vi "ProjektKoncowy.vi"() -> ()   [LabVIEW 2022 SP3]
doc: "Use this template to build a standard state machine design pattern. Each state executes code and determines which state to transition to. Contrast this design pattern with the User Interface Event Handler pattern, in which code executes in response to user actions. Contrast this design pattern also with the Queued Message Handler pattern, in which each message handling code can queue zero or more new messages.\nNote: This template does not contain the most recent programming guidelines recommended by National Instruments. For a complete, project-based implementation of the Standard State Machine pattern, use the Create Project dialog box instead of this template."
uses:
  ProjektKoncowy.ctl
  <vilib>/numeric/Random Number (Range) DBL.vi
  <vilib>/Instr/_visa.llb/VISA Configure Serial Port (Instr).vi
panel:
  in  "Przeskok":dbl(slide)=2.9591836734693877 scale=0.0..10.0
  in  "Szerokosc sciezki":dbl(slide)=5.0 scale=0.0..10.0
  out "Wynik w Grze":dbl
  in  "Stop Button":bool
  out "Gra":waveform(dbl)[](graph)
  out "Dystans w cm":string
  # "Poziom Trudnosci"
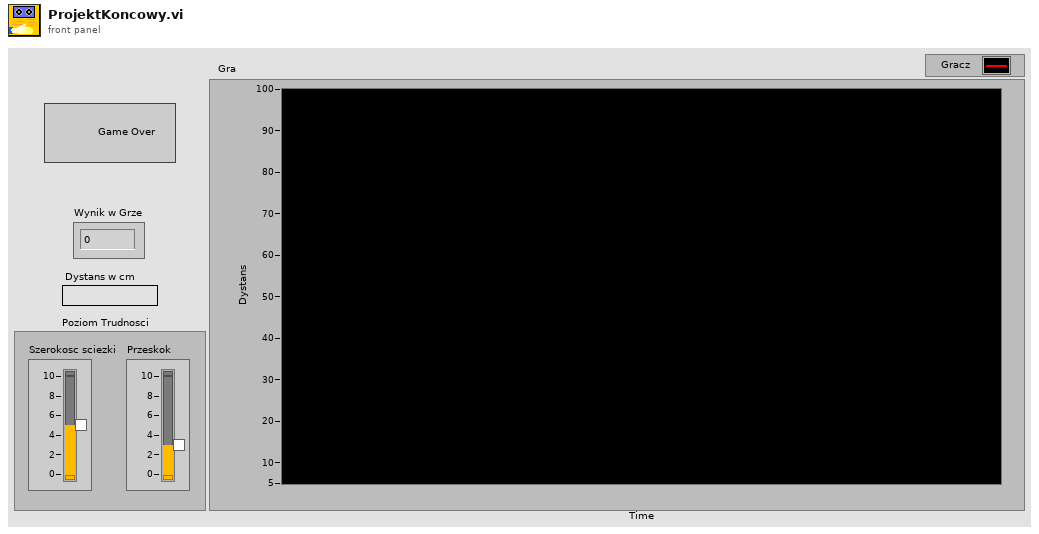
[diagram p1: front panel]
types:
  T1 = typedef "ProjektKoncowy.ctl" = enum16{"Rysuj", "Initialize", "Czytaj dystans", "Stop"}
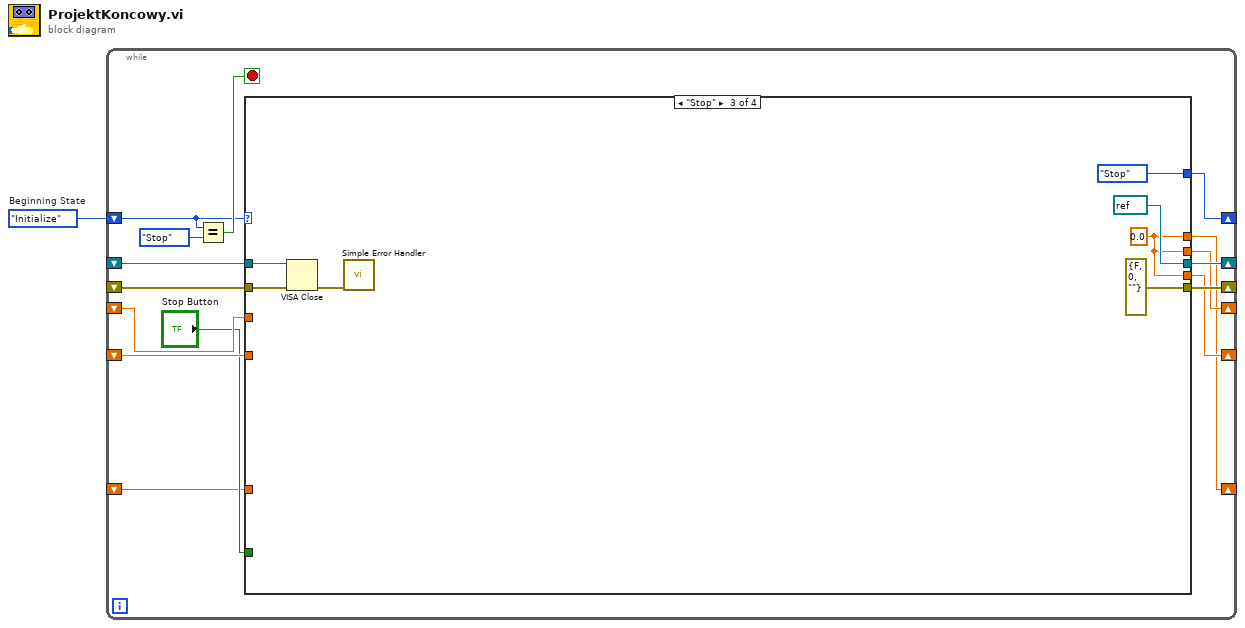
[diagram p0: block diagram]
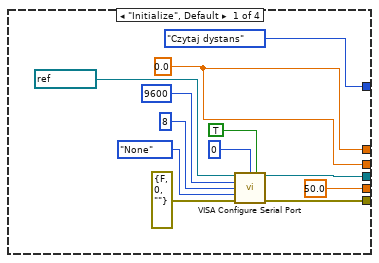
[diagram p2: hidden frame]
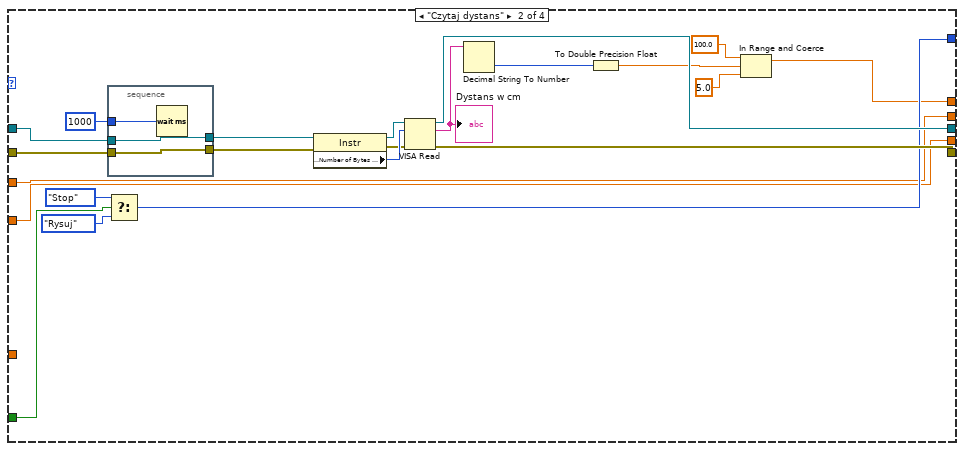
[diagram p3: hidden frame]
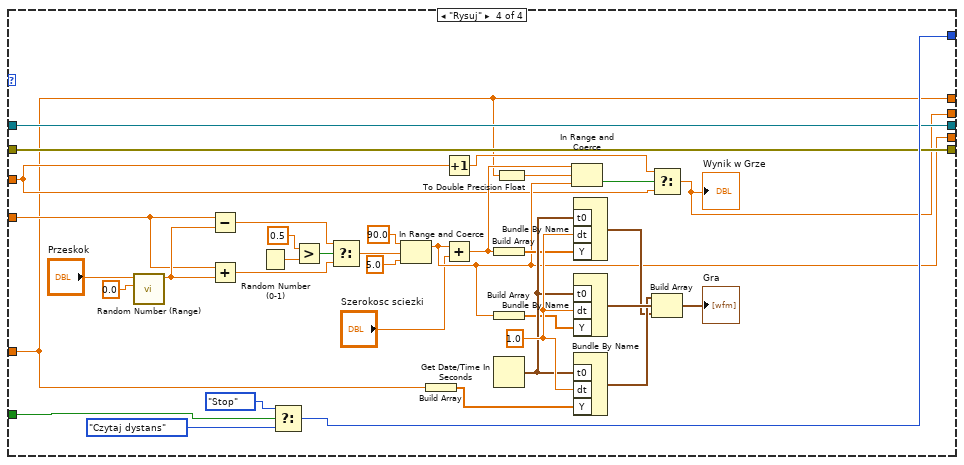
[diagram p4: hidden frame]
diagram:
  w1 = ProjektKoncowy."Initialize"  # Beginning State
  n1 = while {
    shift-right: [w13] -> _
    shift-left: w1 -> [w14]
    shift-right: [w11] -> _
    shift-left: _ -> [w10]
    shift-right: [w12] -> _
    shift-left: _ -> [w9]
    shift-right: [w8] -> _
    shift-left: _ -> [w7]
    shift-right: [w5] -> _
    shift-left: _ -> [w6]
    shift-right: [w3] -> _
    shift-left: _ -> [w2]
    stop <- w16 stop-if-true
    n2 = Equal?(x=w14, y=ProjektKoncowy."Stop" ("States")) -> (x = y?=w16:bool)
    n3 = case shown="\"Stop\"" w14 {
      tunnel: [ProjektKoncowy."Czytaj dystans" ("Next State") w38 ProjektKoncowy."Stop" ("Next State") w94] -> w13
      tunnel: [w28 w50 errorcluster {"status"=FALSE, "code"=0, "source"=""} ("error out") w92] -> w12
      tunnel: [w27 w48 refnum<visa-resource-name> refnum ("VISA resource name out") w91] -> w11
      tunnel: w10 -> [_ w44 w56 w91]
      tunnel: w9 -> [_ w42 w55 w92]
      tunnel: "Stop Button" -> [_ w41 _ w93]
      tunnel: [50.0 ("number") w36 w54 w71] -> w8
      tunnel: w7 -> [_ w36 _ w79]
      tunnel: w6 -> [_ w35 _ w67]
      tunnel: [w17 w35 w54 w64] -> w5
      tunnel: [w17 w29 w54 w61] -> w3
      tunnel: w2 -> [_ _ _ w61]
      frame "Initialize", Default {
        w17 = 0.0
        n4 = call-poly "VISA Configure Serial Port"("VISA resource name"=refnum<visa-resource-name> "COM3", "termination char\n(0xA = '\\n' = LF)"=u8 0 ("termination char\n(0xA = '\\n' = LF)"), "Enable Termination\nChar (T)"=TRUE ("Enable Termination\nChar (T)"), "baud rate (9600)"=u32 9600, "data bits (8)"=u16 8, "parity (0:none)"=enum16{"None", "Odd", "Even", "Mark", "Space"}."None", "error in (no error)"=errorcluster {"status"=FALSE, "code"=0, "source"=""}) -> ("VISA resource name out"=w27:refnum<visa-resource-name>, "error out"=w28:errorcluster)  [unwired: 3 in, 4 out]
      }
      frame "Czytaj dystans" {
        n5 = stacked-sequence {
          tunnel: [w53] -> w45
          tunnel: w44 -> [w53]
          tunnel: [w52] -> w43
          tunnel: w42 -> [w52]
          tunnel: u32 1000 ("Delay (ms)") -> [w51]
          frame #0 {
            n6 = Wait (ms)(milliseconds to wait=w51) -> ()  [unwired: 1 out]
          }
        }
        n7 = Select(t=ProjektKoncowy."Stop", s=w41, f=ProjektKoncowy."Rysuj" ("Next State")) -> (s? t:f=w38:T1)
        n8 = property class="Instr"(reference=w45, error in=w43) -> (reference out=w46:refnum<visa-resource-name>, error out=w47:errorcluster, "Serial Settings:Number of Bytes at Serial Port"=w49:u32)
        n9 = VISA Read(VISA resource name=w46, byte count=w49, error in (no error)=w47) -> (VISA resource name out=w48:refnum<visa-resource-name>, read buffer=w34:string, error out=w50:errorcluster)  [unwired: 1 out]
        "Dystans w cm" <- w34
        n10 = Decimal String To Number(string=w34) -> (number=w33:i32)  [unwired: 2 in, 1 out]
        n11 = To Double Precision Float(number=w33) -> (double precision float=w32:dbl)
        n12 = In Range and Coerce(upper limit=100.0, x=w32, lower limit=5.0) -> (coerced(x)=w29:dbl)  [unwired: 1 out]
      }
      frame "Stop" {
        w54 = 0.0 ("number")
        n13 = VISA Close(VISA resource name=w56, error in (no error)=w55) -> (error out=w57:errorcluster)
        n14 = call <vilib>:"Simple Error Handler.vi"("error in (no error)"=w57) -> ()  [unwired: 1 in, 8 out]
      }
      frame "Rysuj" {
        w87 = 1.0 ("dt")
        n15 = call-poly <vilib>:"Random Number (Range).vi"("lower bound (0)"=0.0, "upper bound (100)"="Przeskok") -> ("number"=w80:dbl)  [unwired: 9 in]
        n16 = Subtract(x=w79, y=w80) -> (x-y=w78:dbl)
        n17 = Add(x=w79, y=w80) -> (x+y=w77:dbl)
        n18 = Random Number (0-1)() -> (number: 0 to 1=w83:dbl)
        n19 = Select(t=ProjektKoncowy."Stop", s=w93, f=ProjektKoncowy."Czytaj dystans" ("Next State")) -> (s? t:f=w94:T1)
        n20 = Greater?(x=0.5, y=w83) -> (0:w81:bool)
        n21 = Select(t=w78, s=w81, f=w77) -> (s? t:f=w73:dbl)
        n22 = In Range and Coerce(upper limit=90.0, x=w73, lower limit=5.0) -> (coerced(x)=w71:dbl)  [unwired: 1 out]
        n23 = Build Array(w61) -> (w62:dbl[])
        n24 = Increment(x=w67) -> (x+1=w68:dbl)
        n25 = Add(x=w71, y="Szerokosc sciezki") -> (x+y=w70:dbl)
        n26 = Build Array(w70) -> (w76:dbl[])
        n27 = Build Array(w71) -> (w72:dbl[])
        n28 = Get Date/Time In Seconds() -> (seconds since 1Jan1904=w84:timestamp)
        n29 = To Double Precision Float(number=w61) -> (double precision float=w63:dbl)
        n30 = In Range and Coerce(upper limit=w70, x=w63, lower limit=w71) -> (In Range?=w69:bool)  [unwired: 1 out]
        n31 = Bundle By Name("t0"=w84, "dt"=w87, "Y"=w76) -> (w86:waveform(dbl))  [unwired: 1 in]
        n32 = Bundle By Name("t0"=w84, "dt"=w87, "Y"=w72) -> (w90:waveform(dbl))  [unwired: 1 in]
        n33 = Bundle By Name("t0"=w84, "dt"=w87, "Y"=w62) -> (w89:waveform(dbl))  [unwired: 1 in]
        n34 = Select(t=w68, s=w69, f=w67) -> (s? t:f=w64:dbl)
        "Wynik w Grze" <- w64
        n35 = Build Array(w89, w90, w86) -> (→"Gra":waveform(dbl)[])
      }
    }
  }
